vi "Global_VS_ref.vi"() -> ()   [LabVIEW 2017]
panel:
  in  "Feedback Section Name":string="O2SensoSim Feedback"
  in  "Control Section Name":string="Additional Control"
  in  "Setpoint Section Name":string="O2SensoSim Setpoint"
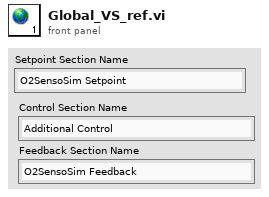
[diagram p1: front panel]
diagram:
